vi "ma_SML Data Packing.vi"   [LabVIEW 2020, in "NI_MAPro.lvlib"]
uses:
  NI_MAPro.lvlib
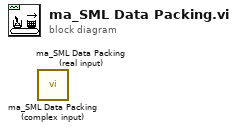
[diagram p0: block diagram]
diagram:
  n1 = call "ma_SML Data Packing (complex input).vi"() -> ()  [unwired: 9 in, 3 out]
  n2 = call "ma_SML Data Packing (real input).vi"() -> ()  [unwired: 9 in, 3 out]
